vi "Saving as CSV files.vi"(0 "First header":string[][](array[string])=[["Fs", "Number of channels"]], 5 "Data Parameters":dbl[](array[numeric]), 7 "Second header":string[][](array[string])=[["Fs", "Number of channels"]], 9 "Timer data":string[][](array[string]), 12 "Third header":string[][](array[string])=[["Fs", "Number of channels"]], 13 "Curve Data":dbl[][](array[numeric])) -> ()   [LabVIEW 2010]
uses:
  <vilib>/Utility/file.llb/Write To Spreadsheet File (string).vi
  <vilib>/Utility/file.llb/Write To Spreadsheet File (DBL).vi
panel:
  out "Image Number":u32
  out "Frame Rate":dbl
  out "FFT angles":dbl[](graph)
  out "FFT Y":dbl[](graph)
  out "FFT X":dbl[](graph)
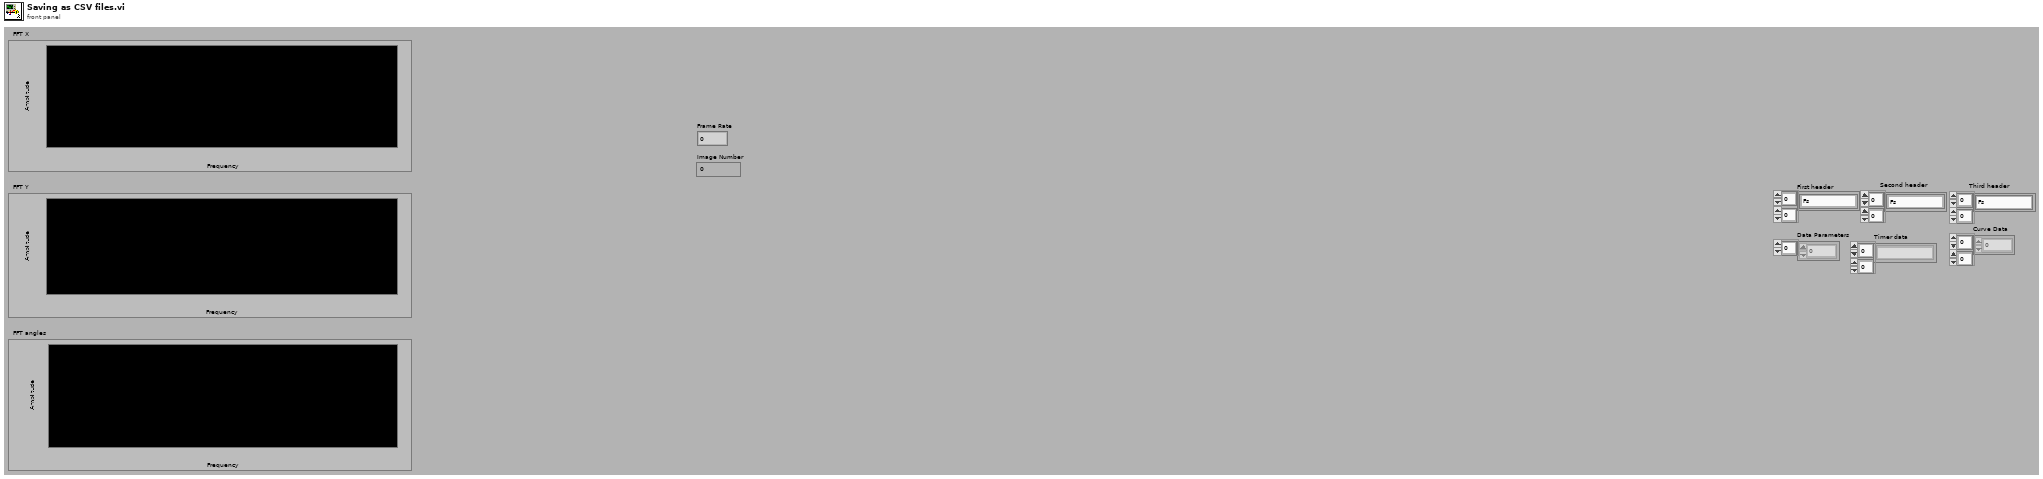
[diagram p1: front panel]
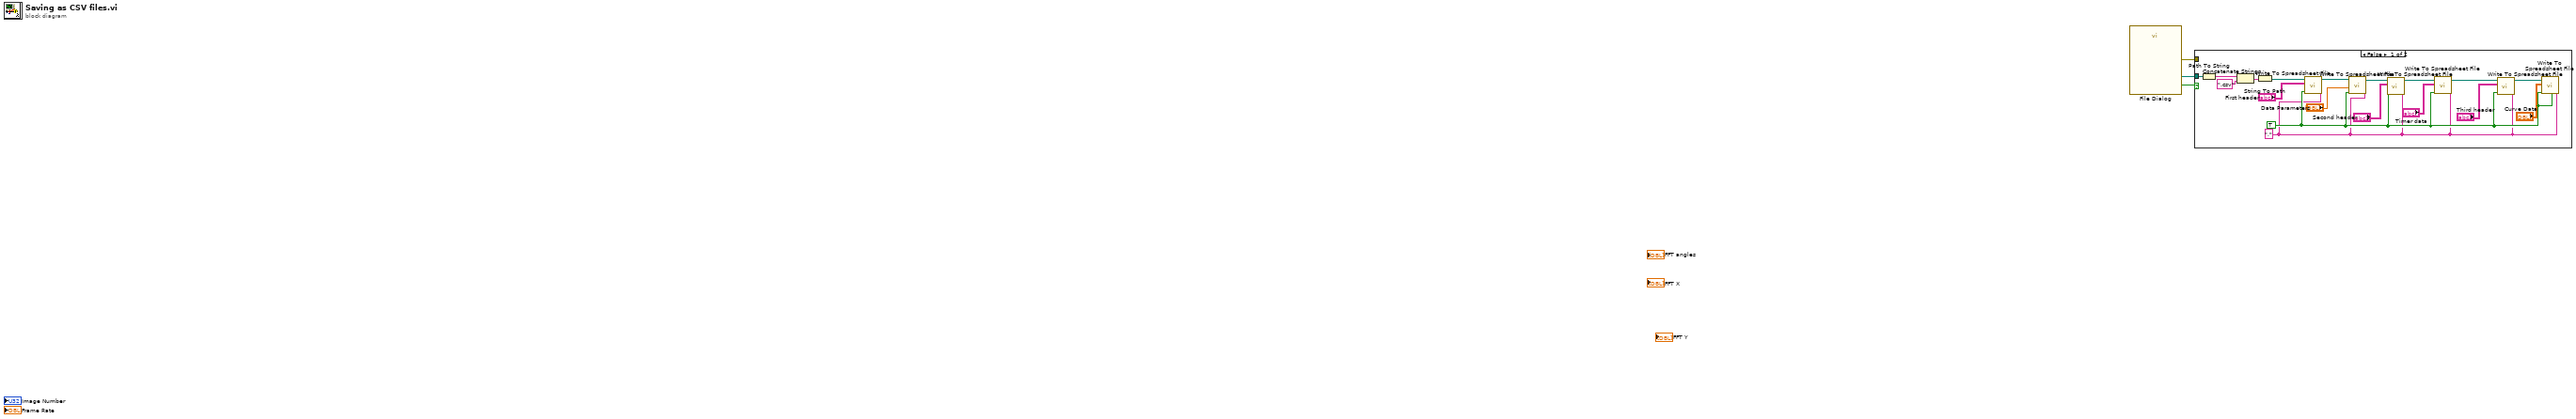
[diagram p0: block diagram]
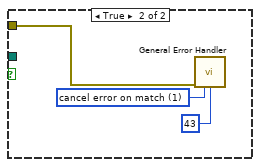
[diagram p2: hidden frame]
diagram:
  n1 = call "File Dialog"() -> ("selected path"=w3:path, "cancelled"=w2:bool, "error out"=w1:errorcluster)  [unwired: 12 in, 1 out]
  n2 = case shown="False" w2 {
    tunnel: w3 -> [w18 _]
    tunnel: w1 -> [_ w24]
    frame False {
      w5 = "," ("delimiter (\\t)")
      w6 = TRUE ("append to file? (new file:F)")
      n3 = Path To String(path=w18) -> (string=w17:string)
      n4 = Concatenate Strings(w17, ".csv" ("string")) -> (w16:string)
      n5 = String To Path(string=w16) -> (path=w15:path)
      n6 = call-poly <vilib>:"Write To Spreadsheet File.vi"("delimiter (\\t)"=w5, "append to file? (new file:F)"=w6, "2D data"="First header", "file path (dialog if empty)"=w15) -> ("new file path (Not A Path if cancelled)"=w19:path)  [unwired: 4 in]
      n7 = call-poly <vilib>:"Write To Spreadsheet File.vi"("delimiter (\\t)"=w5, "append to file? (new file:F)"=w6, "1D data"="Data Parameters", "file path (dialog if empty)"=w19) -> ("new file path (Not A Path if cancelled)"=w9:path)  [unwired: 4 in]
      n8 = call-poly <vilib>:"Write To Spreadsheet File.vi"("delimiter (\\t)"=w5, "append to file? (new file:F)"=w6, "2D data"="Second header", "file path (dialog if empty)"=w9) -> ("new file path (Not A Path if cancelled)"=w8:path)  [unwired: 4 in]
      n9 = call-poly <vilib>:"Write To Spreadsheet File.vi"("delimiter (\\t)"=w5, "append to file? (new file:F)"=w6, "2D data"="Timer data", "file path (dialog if empty)"=w8) -> ("new file path (Not A Path if cancelled)"=w7:path)  [unwired: 4 in]
      n10 = call-poly <vilib>:"Write To Spreadsheet File.vi"("delimiter (\\t)"=w5, "append to file? (new file:F)"=w6, "2D data"="Third header", "file path (dialog if empty)"=w7) -> ("new file path (Not A Path if cancelled)"=w21:path)  [unwired: 4 in]
      n11 = call-poly <vilib>:"Write To Spreadsheet File.vi"("delimiter (\\t)"=w5, "transpose? (no:F)"=w6, "append to file? (new file:F)"=w6, "2D data"="Curve Data", "file path (dialog if empty)"=w21) -> ()  [unwired: 3 in, 1 out]
    }
    frame True {
      w22 = 1 items=["no exception", "cancel error on match", "set error on match"] ("[exception action] (none:0)")
      n12 = call <vilib>:"General Error Handler.vi"("error in (no error)"=w24, "[exception action] (none:0)"=w22, "[exception code]"=43) -> ()  [unwired: 8 in, 5 out]
    }
  }
